vi "StartExecutionCallback.vi"(4 "User Parameter":variant, 5 "Event Data":T1, 6 "Control Ref":refnum<k7>, 7 "Event Common Data":T2) -> ()   [LabVIEW 2010]
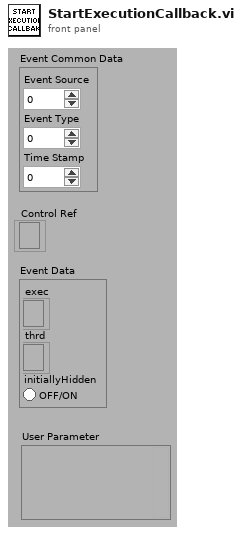
[diagram p1: front panel]
types:
  T1 = cluster{"exec":refnum<k7>, "thrd":refnum<k7>, "initiallyHidden":bool}
  T2 = cluster{"Event Source":i32, "Event Type":u32, "Time Stamp":u32}
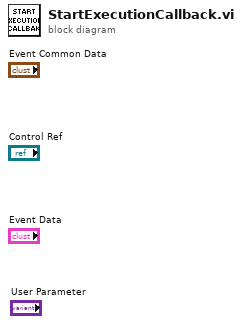
[diagram p0: block diagram]
diagram:
